vi "Close Config Data.vi"(8 "error in (no error)":errorcluster caption="Fehler (Eingang, kein Fehler)", 10 "write configuration file? (T)":bool=TRUE caption="Konfigurationsdaten schreiben? (T)", 11 "refnum":T1 caption="RefNum") -> (0 "error out":errorcluster caption="Fehler (Ausgang)")   [LabVIEW 2009]
doc: "Beendet eine durch <B>Refnum</B> angegebene Referenz zu einer Konfigurationsdatei."
uses:
  <vilib>/Utility/config.llb/Config Data RefNum.ctl
  <vilib>/Utility/config.llb/NI_LVConfig.lvlib
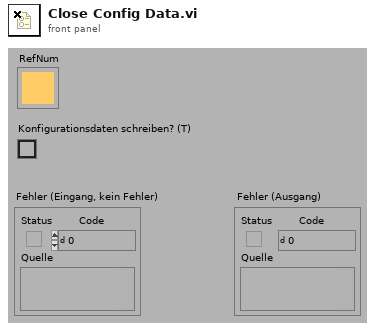
[diagram p1: front panel]
types:
  T1 = typedef "NI_LVConfig.lvlib/Config Data RefNum.ctl" = refnum<k1>
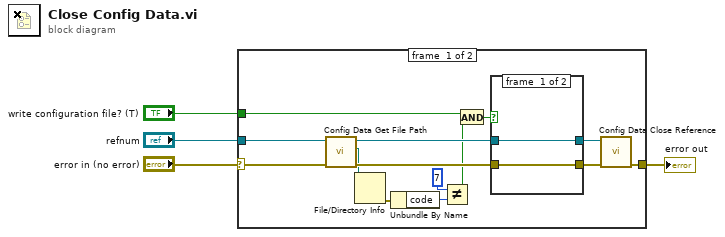
[diagram p0: block diagram]
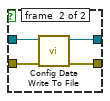
[diagram p2: hidden frame]
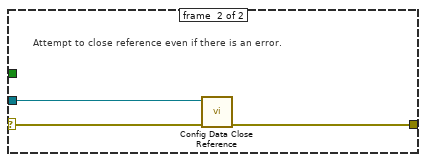
[diagram p3: hidden frame]
diagram:
  n1 = case shown="No Error" "error in (no error)" {
    selector: "error in (no error)" -> [w5 w25]
    tunnel: [w17 w27] -> w4
    tunnel: "refnum" -> [w7 w26]
    tunnel: "write configuration file? (T)" -> [w9 _]
    frame #0 {
      n2 = call "Config Data Get File Path.vi"("error in (no error)"=w5, "config data reference"=w7) -> ("error out"=w16:errorcluster, "file path"=w14:path, "config data reference out"=w15:T1)  [unwired: 7 in]
      n3 = File/Directory Info(path=w14) -> (error out=w13:errorcluster)  [unwired: 1 in, 6 out]
      n4 = Unbundle By Name(w13) -> ("code"=w12:i32)
      n5 = Not Equal?(x=7 ("code"), y=w12) -> (x != y?=w10:bool)
      n6 = And(x=w9, y=w10) -> (x .and. y?=w8:bool)
      n7 = case shown="True" w8 {
        tunnel: w16 -> [w19 w24]
        tunnel: w15 -> [w20 w23]
        tunnel: [w19 w22] -> w6
        tunnel: [w20 w21] -> w18
        frame #0 {
        }
        frame #1 {
          n8 = call "Config Data Write To File.vi"("error in (no error)"=w24, "config data reference"=w23) -> ("error out"=w22:errorcluster, "config data reference out"=w21:T1)  [unwired: 8 in]
        }
      }
      n9 = call "Config Data Close Reference.vi"("error in (no error)"=w6, "config data reference"=w18) -> ("error out"=w17:errorcluster)  [unwired: 9 in]
    }
    frame #1 {
      # "Attempt to close reference even if there is an error."
      n10 = call "Config Data Close Reference.vi"("error in (no error)"=w25, "config data reference"=w26) -> ("error out"=w27:errorcluster)  [unwired: 9 in]
    }
  }
  "error out" <- w4
